vi "Do.vi"(8 "error in (no error)":errorcluster, 10 "Actor in":refnum<class "Actor.lvclass">, 11 "Goto Msg":refnum<class "Goto Msg.lvclass">) -> (0 "error out":errorcluster, 2 "Actor out":refnum<class "Actor.lvclass">)   [LabVIEW 2023, in "Goto Msg.lvclass"]
doc: "This VI delivers the message to the actor by calling the appropriate method(s) on the actor."
uses:
  Goto Msg.lvclass
  Goto Msg.lvclass/Goto Msg.ctl
  9ef47adc-f318-494c-9b8b-6df3216d6863.vi
  TranslationStages/TranslationStages.lvclass
  <vilib>/ActorFramework/Actor/Actor.lvclass
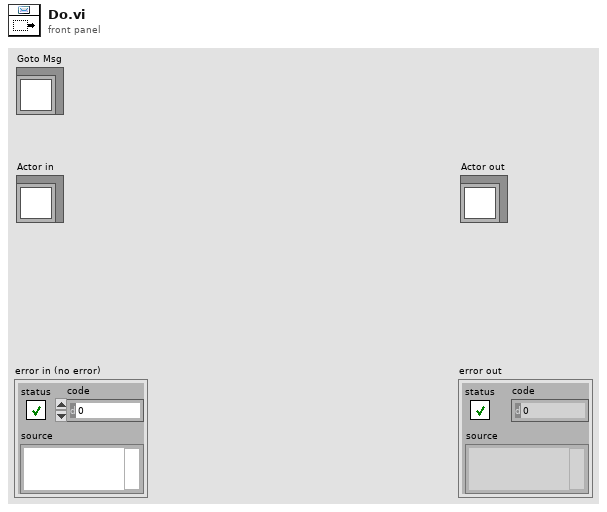
[diagram p1: front panel]
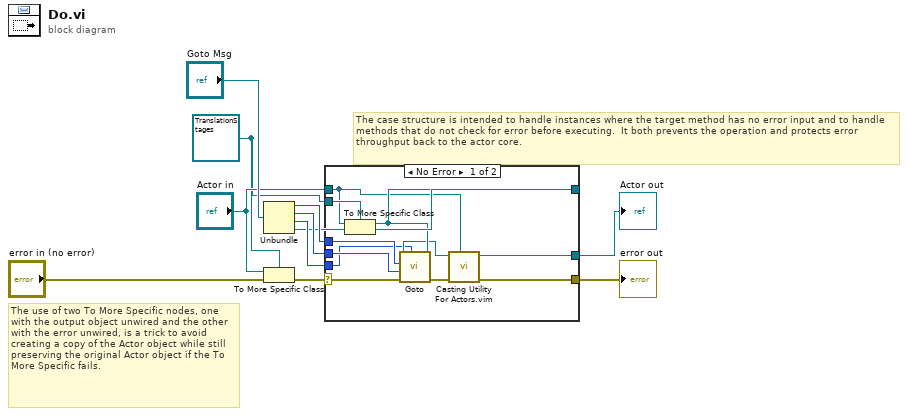
[diagram p0: block diagram]
diagram:
  w5 = refnum<class "TranslationStages.lvclass"> refnum ("Actor in")
  # "The use of two To More Specific nodes, one with the output object unwired and the other with the error unwired, is a trick to avoid creating a copy of the Actor object while still preserving the original Actor object if the To More Specific fails."
  # "The case structure is intended to handle instances where the target method has no error input and to handle methods that do not check for error before executing.  It both prevents the operation and protects error throughput back to the actor core."
  n1 = Unbundle("Goto Msg") -> (w4:enum16{""}, w3:enum16{""}, w2:i32, w1:refnum<class "TranslationStages.lvclass">)
  n2 = To More Specific Class(target class=w5, reference="Actor in", error in="error in (no error)") -> (error out=w9:errorcluster)  [unwired: 1 out]
  n3 = case shown="No Error" w9 {
    selector: w9 -> [w22 w24]
    tunnel: [w16 w24] -> w8
    tunnel: [w17 w23] -> w7
    tunnel: "Actor in" -> [w19 w23]
    tunnel: w5 -> [w20 _]
    tunnel: w4 -> [w14 _]
    tunnel: w3 -> [w13 _]
    tunnel: w2 -> [w12 _]
    tunnel: w1 -> [w21 _]
    frame No Error {
      n4 = To More Specific Class(target class=w20, reference=w19) -> (specific class reference=w21:refnum<class "TranslationStages.lvclass">)  [unwired: 1 in, 1 out]
      n5 = call "Goto.vi"("TranslationStages.lvclass"=w21, "Speed"=w12, "error in (no error)"=w22, "Direction"=w13, "New Position"=w14) -> ("error out"=w15:errorcluster, "TranslationStages.lvclass"=w18:refnum<class "TranslationStages.lvclass">)  [unwired: 5 in]
      n6 = call "Casting Utility For Actors.vim"("type"=w19, "error in (no error)"=w15, "Actor in"=w18) -> ("error out"=w16:errorcluster, "Actor out"=w17:refnum<class "Actor.lvclass">)  [unwired: 7 in]
    }
    frame Error {
      # "If type check fails, pass the original object out again."
    }
  }
  "error out" <- w8
  "Actor out" <- w7
